vi "Flatten To JSON String.vi"(4 "Enums As String (F)":bool, 5 "Numeric Extensions (F)":bool, 6 "Timestamp Options":T1={"Convert Timestamps"=TRUE, "UTC"=TRUE}, 7 "Multiline (T)":bool=TRUE, 8 "error in (no error)":errorcluster, 11 "Variant":variant) -> (0 "error out":errorcluster, 3 "JSON String":string)   [LabVIEW 2020, in "JKI JSON Serialization.lvlib"]
doc: "Converts <b>Variant</b> to <b>JSON String</b>. If <b>Multiline</b> is false returns a single-line JSON string, otherwise returns a pretty-printed multi-line string. If <b>Numeric Extensions</b> is true, converts +-Inf and NaN to symbolic values compatible with many JSON libraries but not part of JSON standard. If <b>Convert Timestamps</b> is true in <b>Timestamp Options</b> converts LabVIEW timestamps to ISO timestamp strings. If <b>UTC</b>is true, uses universal time instead of local time."
uses:
  JKI JSON Serialization.lvlib
  Timestamp Options.ctl
  Serializer/JSON Serializer/JSON Serializer.lvclass
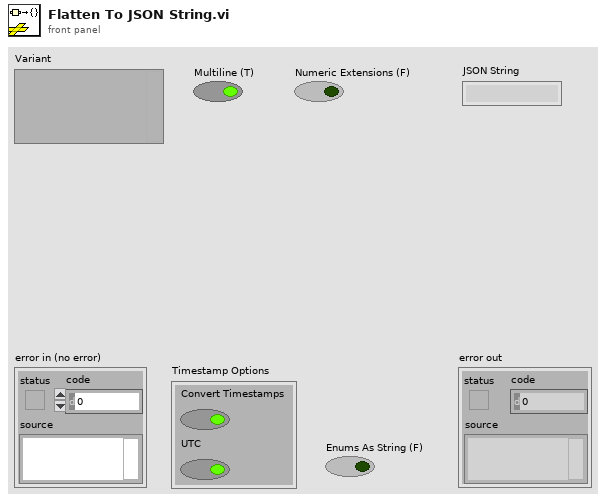
[diagram p1: front panel]
types:
  T1 = typedef "JKI JSON Serialization.lvlib/Timestamp Options.ctl" = cluster{"Convert Timestamps":bool, "UTC":bool}
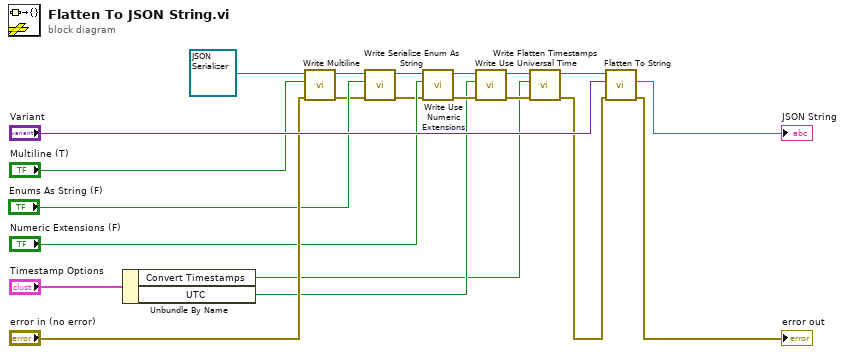
[diagram p0: block diagram]
diagram:
  n1 = Unbundle By Name("Timestamp Options") -> ("Convert Timestamps"=w6:bool, "UTC"=w7:bool)
  n2 = call-dynamic "Write Multiline.vi"("error in (no error)"="error in (no error)", "Multiline"="Multiline (T)", "JSON Serializer in"=refnum<class "JSON Serializer.lvclass"> refnum) -> ("error out"=w3:errorcluster, "JSON Serializer out"=w5:refnum<class "JSON Serializer.lvclass">)  [unwired: 7 in]
  n3 = call-dynamic "Write Serialize Enum As String.vi"("error in (no error)"=w3, "Enums As String"="Enums As String (F)", "JSON Serializer in"=w5) -> ("error out"=w2:errorcluster, "JSON Serializer out"=w1:refnum<class "JSON Serializer.lvclass">)  [unwired: 7 in]
  n4 = call-dynamic "Write Use Numeric Extensions.vi"("error in (no error)"=w2, "Numeric Extensions"="Numeric Extensions (F)", "JSON Serializer in"=w1) -> ("error out"=w15:errorcluster, "JSON Serializer out"=w16:refnum<class "JSON Serializer.lvclass">)  [unwired: 7 in]
  n5 = call-dynamic "Write Use Universal Time.vi"("error in (no error)"=w15, "Universal Time"=w7, "JSON Serializer in"=w16) -> ("error out"=w14:errorcluster, "JSON Serializer out"=w18:refnum<class "JSON Serializer.lvclass">)  [unwired: 7 in]
  n6 = call-dynamic "Write Flatten Timestamps.vi"("error in (no error)"=w14, "Convert Timestamps"=w6, "JSON Serializer in"=w18) -> ("error out"=w12:errorcluster, "JSON Serializer out"=w11:refnum<class "JSON Serializer.lvclass">)  [unwired: 7 in]
  n7 = call-dynamic "Flatten To String.vi"("error in (no error)"=w12, "Variant"="Variant", "JSON Serializer in"=w11) -> ("error out"=→"error out":errorcluster, "String"=→"JSON String":string)  [unwired: 6 in, 1 out]
